vi "Mask Write Holding Register.vi"(4 "OR mask":u16, 6 "AND mask":u16, 8 "error in (no error)":errorcluster, 10 "address":u16, 11 "Modbus master in":refnum<class "Modbus Master.lvclass">) -> (0 "error out":errorcluster, 3 "Modbus master out":refnum<class "Modbus Master.lvclass">)   [LabVIEW 2021, in "Modbus Master.lvclass"]
doc: "Writes values to one or more bits of a holding register."
uses:
  Modbus Master.lvclass
  Modbus Master.lvclass/Modbus Master.ctl
  Master Function Definition/Master Function Definition.lvclass
  Network Protocol/Network Master/Network Master.lvclass
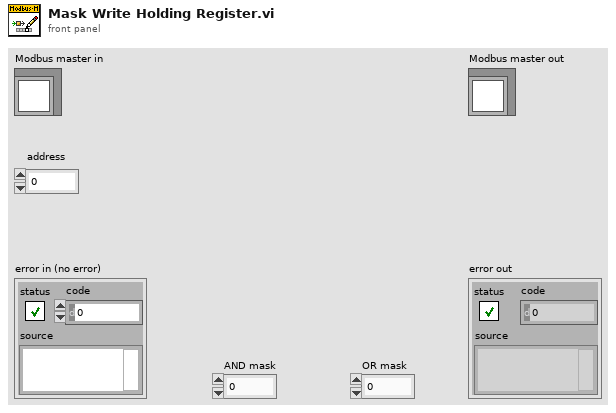
[diagram p1: front panel]
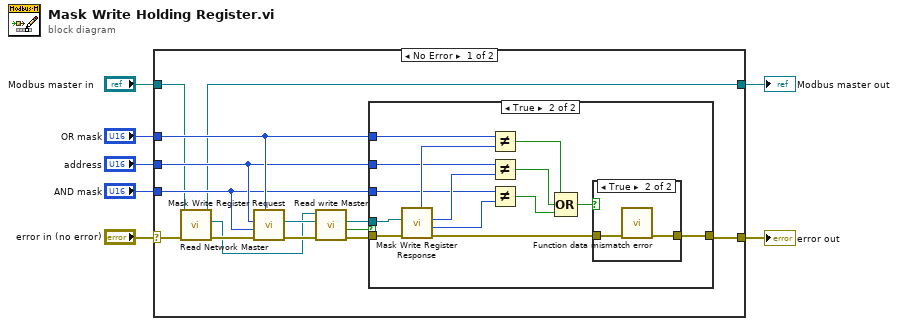
[diagram p0: block diagram]
diagram:
  n1 = case shown="No Error" "error in (no error)" {
    selector: "error in (no error)" -> [w14 w40]
    tunnel: "Modbus master in" -> [w15 w41]
    tunnel: [w8 w41] -> w6
    tunnel: [w20 w40] -> w5
    tunnel: "OR mask" -> [w18 _]
    tunnel: "address" -> [w17 _]
    tunnel: "AND mask" -> [w16 _]
    frame No Error {
      n2 = call "Read Network Master.vi"("error in"=w14, "Modbus master in"=w15) -> ("error out"=w13:errorcluster, "Network Master"=w11:refnum<class "Network Master.lvclass">, "Modbus master out"=w8:refnum<class "Modbus Master.lvclass">)  [unwired: 7 in]
      n3 = call "Mask Write Register Request.vi"("OR mask"=w18, "error in"=w13, "AND mask"=w16, "Starting Address"=w17) -> ("error out"=w21:errorcluster, "modbus data unit out"=w12:refnum<class "Modbus Data Unit.lvclass">)  [unwired: 6 in]
      n4 = call "Read write Master.vi"("error in (no error)"=w21, "Modbus data unit in"=w12, "Modbus master in"=w11) -> ("error out"=w19:errorcluster, "PDU valid?"=w10:bool, "Modbus data unit out"=w9:refnum<class "Modbus Data Unit.lvclass">)  [unwired: 5 in, 1 out]
      n5 = case shown="True" w10 {
        tunnel: [w22 w34] -> w20
        tunnel: w19 -> [w22 w31]
        tunnel: w9 -> [_ w30]
        tunnel: w18 -> [_ w25]
        tunnel: w16 -> [_ w24]
        tunnel: w17 -> [_ w23]
        frame False {
        }
        frame True {
          n6 = call "Mask Write Register Response.vi"("error in"=w31, "modbus data unit in"=w30) -> ("error out"=w29:errorcluster, "AND mask"=w32:u16, "Address"=w33:u16, "OR mask"=w26:u16)  [unwired: 6 in]
          n7 = Not Equal?(x=w25, y=w26) -> (x != y?=w27:bool)
          n8 = Not Equal?(x=w23, y=w33) -> (x != y?=w28:bool)
          n9 = Not Equal?(x=w24, y=w32) -> (x != y?=w36:bool)
          n10 = Compound Arithmetic op=OR(w27, w28, w36) -> (w35:bool)
          n11 = case shown="True" w35 {
            tunnel: [w37 w39] -> w34
            tunnel: w29 -> [w37 w38]
            frame False {
            }
            frame True {
              n12 = call "Function data mismatch error.vi"("error in (no error)"=w38) -> ("error out"=w39:errorcluster)  [unwired: 10 in]
            }
          }
        }
      }
    }
    frame Error {
    }
  }
  "error out" <- w5
  "Modbus master out" <- w6
